vi "data_write.vi"(8 "error in (no error)":errorcluster, 10 "data":variant, 11 "ini_file_refnum":T1) -> (0 "error out":errorcluster, 3 "ini_file_refnum_out":T1)   [LabVIEW 2015, in "ini_work_Library.lvlib"]
doc: "Created by Artem Shevelev\nshevelev.pro\nartem@shevelev.pro\nLabVIEW Portal: https://labviewportal.org/memberlist.php?mode=viewprofile&u=2340"
uses:
  ini_work_Library.lvlib
  <vilib>/Utility/config.llb/Config Data RefNum.ctl
  <vilib>/Utility/config.llb/NI_LVConfig.lvlib
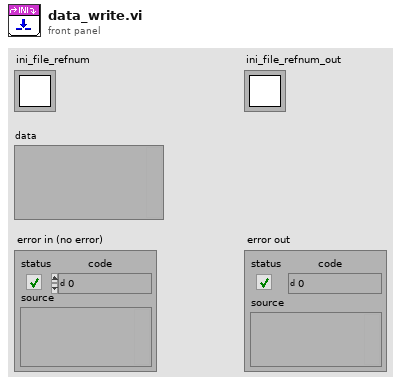
[diagram p1: front panel]
types:
  T1 = typedef "NI_LVConfig.lvlib/Config Data RefNum.ctl" = refnum<k1>
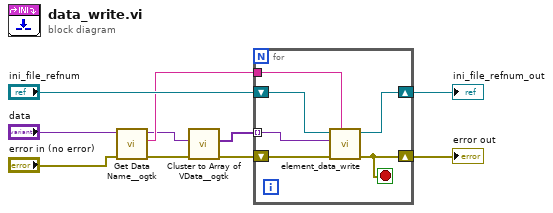
[diagram p0: block diagram]
diagram:
  n1 = call <userlib>:"Get Data Name__ogtk.vi"("error in (no error)"="error in (no error)", "Data"="data") -> ("error out"=w2:errorcluster, "Data Name"=w5:string, "Data dup"=w1:variant)  [unwired: 7 in]
  n2 = call <userlib>:"Cluster to Array of VData__ogtk.vi"("error in (no error)"=w2, "Cluster"=w1) -> ("error out"=w9:errorcluster, "Array of VData"=w10:variant[])  [unwired: 8 in]
  n3 = for {
    tunnel: w10 -> [w11] mode=indexing
    shift-right: [w13] -> w3
    shift-left: w9 -> [w15]
    shift-right: [w14] -> w4
    shift-left: "ini_file_refnum" -> [w16]
    tunnel: w5 -> [w12]
    stop <- w13 stop-if-true
    n4 = call "element_data_write.vi"("container_name"=w12, "error in (no error)"=w15, "Variant"=w11, "Refnum in"=w16) -> ("error out"=w13:errorcluster, "Refnum out"=w14:T1)  [unwired: 6 in]
  }
  "ini_file_refnum_out" <- w4
  "error out" <- w3
